vi "multiply.vi"(10 "String 2":string, 11 "String":string) -> (3 "String 3":string)   [LabVIEW 2025]
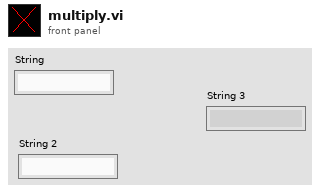
[diagram p1: front panel]
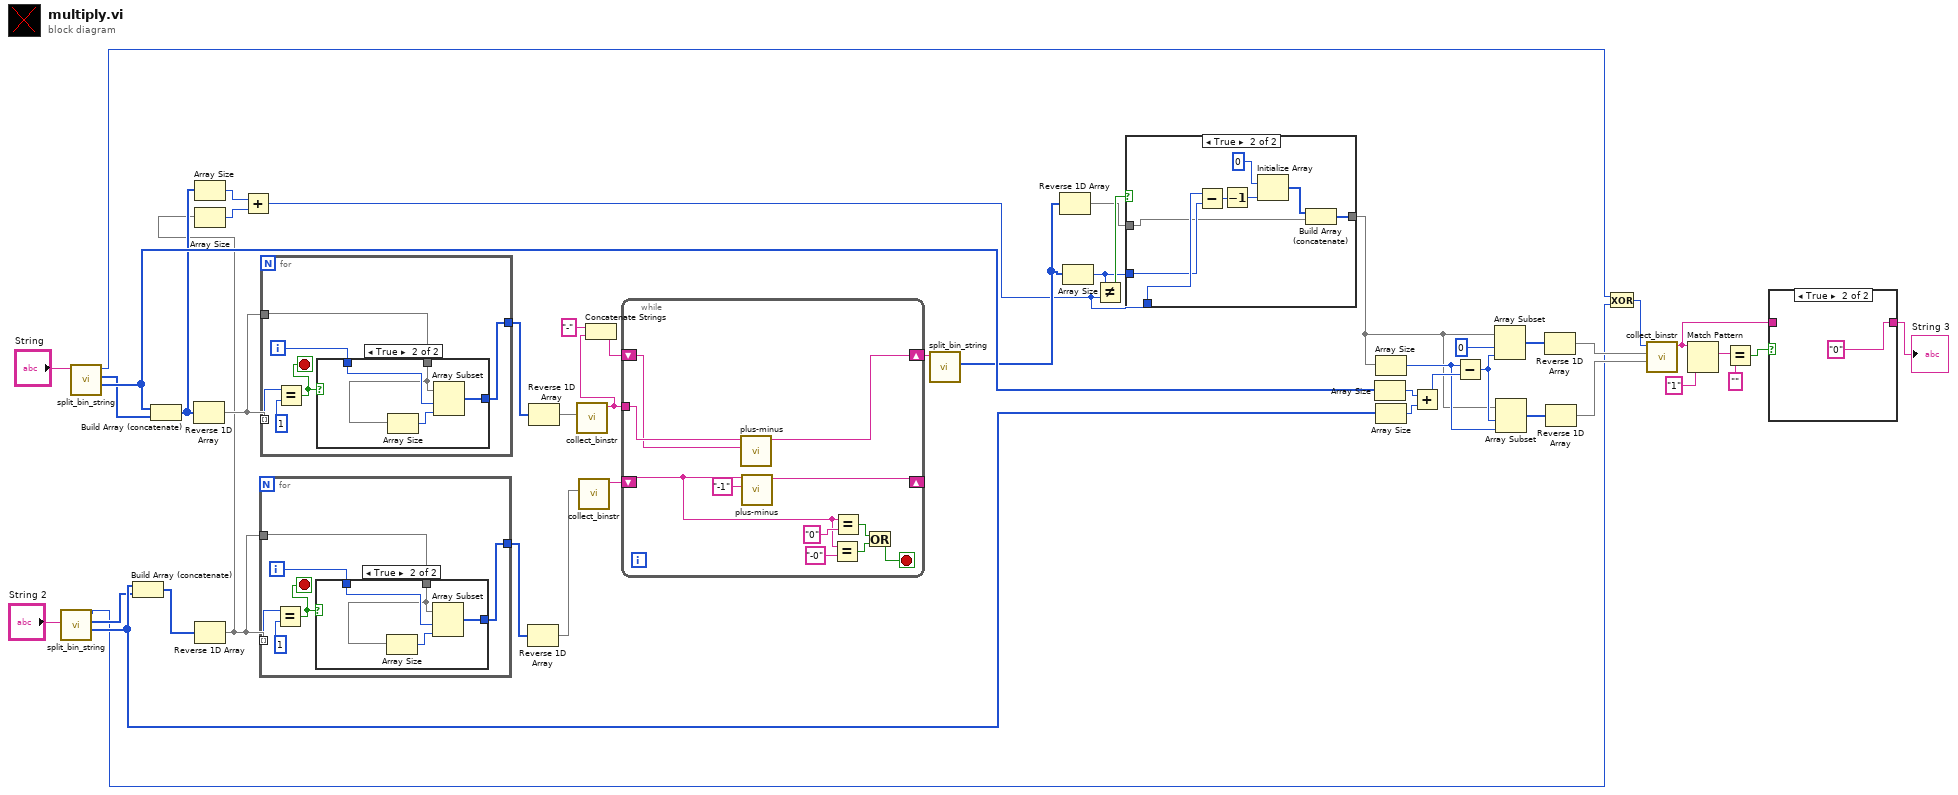
[diagram p0: block diagram]
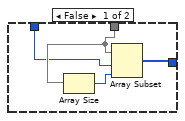
[diagram p4: hidden frame]
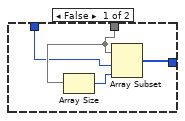
[diagram p5: hidden frame]
diagram:
  n1 = call "split_bin_string.vi"("String"="String 2") -> ("Fraction"=w31:u8[], "Integer"=w30:u8[], "Sign"=w8:u8)  [unwired: 8 in]
  n2 = call "split_bin_string.vi"("String"="String") -> ("Fraction"=w33:u8[], "Integer"=w32:u8[], "Sign"=w9:u8)  [unwired: 8 in]
  n3 = Build Array (concatenate)(w31, w30) -> (w21:u8[])
  n4 = Build Array (concatenate)(w33, w32) -> (w19:u8[])
  n5 = Reverse 1D Array(array=w19) -> (reversed array=w25:u8[])
  n6 = Array Size(array=w19) -> (size(s)=w16:i32)
  n7 = Reverse 1D Array(array=w21) -> (reversed array=w18:u8[])
  n8 = Array Size(array=w18) -> (size(s)=w17:i32)
  n9 = Add(x=w16, y=w17) -> (x+y=w13:i32)
  n10 = for {
    tunnel: w18 -> [w52] mode=indexing
    tunnel: w18 -> [w48]
    tunnel: [w47] -> w22
    i -> [w49]
    stop <- w50 stop-if-true
    n11 = Equal?(x=w52, y=u8 1) -> (x = y?=w50:bool)
    n12 = case shown="True" w50 {
      tunnel: w49 -> [w53 w60]
      tunnel: w48 -> [w56 w59]
      tunnel: [w54 w57] -> w47
      frame False {
        n13 = Array Size(array=w56) -> (size(s)=w55:i32)
        n14 = Array Subset(array=w56, index=w53, length=w55) -> (w54:u8[])
      }
      frame True {
        n15 = Array Size(array=w59) -> (size(s)=w58:i32)
        n16 = Array Subset(array=w59, index=w60, length=w58) -> (w57:u8[])
      }
    }
  }
  n17 = for {
    tunnel: w25 -> [w66] mode=indexing
    tunnel: w25 -> [w62]
    tunnel: [w61] -> w24
    i -> [w63]
    stop <- w64 stop-if-true
    n18 = Equal?(x=w66, y=u8 1) -> (x = y?=w64:bool)
    n19 = case shown="True" w64 {
      tunnel: w63 -> [w67 w74]
      tunnel: w62 -> [w70 w73]
      tunnel: [w68 w71] -> w61
      frame False {
        n20 = Array Size(array=w70) -> (size(s)=w69:i32)
        n21 = Array Subset(array=w70, index=w67, length=w69) -> (w68:u8[])
      }
      frame True {
        n22 = Array Size(array=w73) -> (size(s)=w72:i32)
        n23 = Array Subset(array=w73, index=w74, length=w72) -> (w71:u8[])
      }
    }
  }
  n24 = Reverse 1D Array(array=w22) -> (reversed array=w20:u8[])
  n25 = Reverse 1D Array(array=w24) -> (reversed array=w23:u8[])
  n26 = call "collect_binstr.vi"("Integer"=w23) -> ("String"=w27:string)  [unwired: 10 in]
  n27 = call "collect_binstr.vi"("Integer"=w20) -> ("String"=w29:string)  [unwired: 10 in]
  n28 = Concatenate Strings("-" ("string"), w27) -> (w26:string)
  n29 = while {
    tunnel: w27 -> [w85]
    shift-right: [w83] -> w44
    shift-left: w26 -> [w84]
    shift-right: [w81] -> _
    shift-left: w29 -> [w78]
    stop <- w75 stop-if-true
    n30 = call "plus-minus.vi"("String 2"=w84, "String"=w85) -> ("String 3"=w83:string)  [unwired: 9 in]
    n31 = call "plus-minus.vi"("String 2"="-1", "String"=w78) -> ("String 3"=w81:string)  [unwired: 9 in]
    n32 = Equal?(x=w78, y="-0") -> (x = y?=w77:bool)
    n33 = Equal?(x=w78, y="0") -> (x = y?=w76:bool)
    n34 = Or(x=w76, y=w77) -> (x .or. y?=w75:bool)
  }
  n35 = call "split_bin_string.vi"("String"=w44) -> ("Integer"=w15:u8[])  [unwired: 8 in, 2 out]
  n36 = Reverse 1D Array(array=w15) -> (reversed array=w11:u8[])
  n37 = Array Size(array=w15) -> (size(s)=w12:i32)
  n38 = Not Equal?(x=w12, y=w13) -> (x != y?=w14:bool)
  n39 = case shown="True" w14 {
    tunnel: w13 -> [_ w94]
    tunnel: w12 -> [_ w93]
    tunnel: w11 -> [w86 w90]
    tunnel: [w86 w89] -> w10
    frame False {
    }
    frame True {
      n40 = Subtract(x=w94, y=w93) -> (x-y=w88:i32)
      n41 = Decrement(x=w88) -> (x-1=w87:i32)
      n42 = Initialize Array(u8 0 ("element"), w87) -> (w91:u8[])
      n43 = Build Array (concatenate)(w91, w90) -> (w89:u8[])
    }
  }
  n44 = Array Size(array=w33) -> (size(s)=w42:i32)
  n45 = Array Size(array=w10) -> (size(s)=w38:i32)
  n46 = Array Size(array=w31) -> (size(s)=w41:i32)
  n47 = Add(x=w42, y=w41) -> (x+y=w40:i32)
  n48 = Subtract(x=w38, y=w40) -> (x-y=w39:i32)
  n49 = Array Subset(array=w10, index=0, length=w39) -> (w37:u8[])
  n50 = Array Subset(array=w10, index=w39, length=w38) -> (w35:u8[])
  n51 = Reverse 1D Array(array=w37) -> (reversed array=w36:u8[])
  n52 = Reverse 1D Array(array=w35) -> (reversed array=w34:u8[])
  n53 = Exclusive Or(1:w8, 2:w9) -> (0:w7:u8)
  n54 = call "collect_binstr.vi"("Fraction"=w34, "Integer"=w36, "Sign"=w7) -> ("String"=w2:string)  [unwired: 8 in]
  n55 = Match Pattern(string=w2, regular expression="1") -> (match substring=w5:string)  [unwired: 1 in, 3 out]
  n56 = Equal?(x=w5, y="") -> (x = y?=w3:bool)
  n57 = case shown="True" w3 {
    tunnel: w2 -> [w95 _]
    tunnel: [w95 "0"] -> w1
    frame False {
    }
    frame True {
    }
  }
  "String 3" <- w1
